vi "CarWashTest.vi"(0 "Wash Option":string, 2 "Label":string, 5 "Car Position":u8=1, 7 "Elapsed Time":dbl=5.0, 11 "error in":errorcluster) -> (15 "error out":errorcluster)   [LabVIEW 2016]
uses:
  Car Wash 16.0/Car Wash.vi
  main/apis/Stimulus/ValueSignalByPathString.vi
  main/apis/Assert/AssertControlValueCompare/AssertControlValueEqual.vi
  main/apis/Setup/GetVI/GetVIByPath.vi
  main/apis/Assert/AssertControlValueCompare/AssertControlValueAlmostEqual.vi
  <vilib>/addons/_JKI Toolkits/Caraya/classes/Test/Test.lvclass
  Car Wash 16.0/Car Wash.lvlib
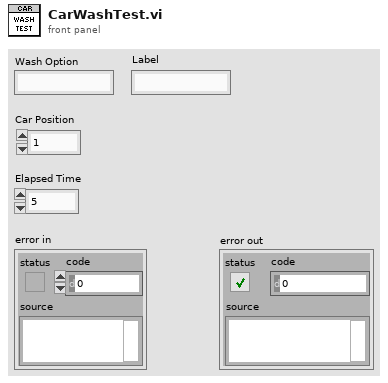
[diagram p1: front panel]
types:
  T1 = enum32{"Invalid", "Standard", "Closed", "Hidden", "Minimized", "Maximized"}
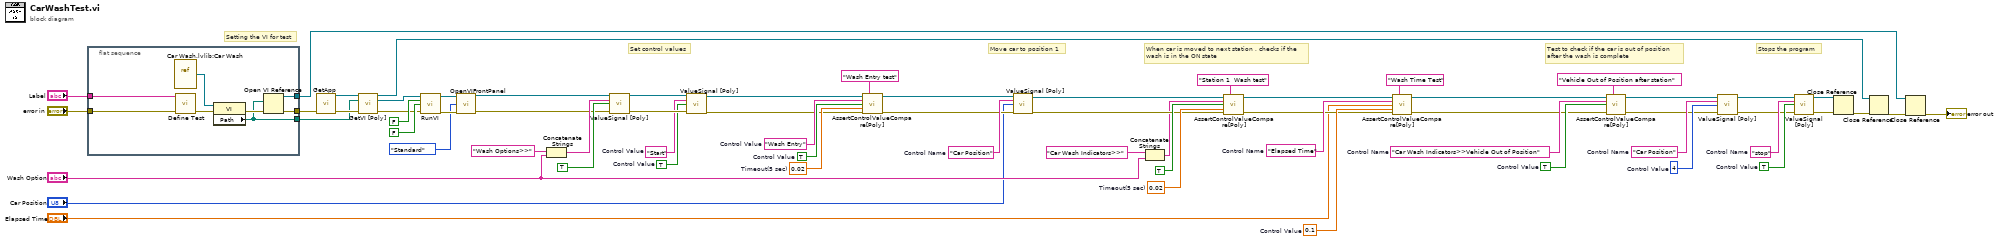
[diagram p0: block diagram]
diagram:
  w11 = TRUE  # Control Value
  w12 = "stop"  # Control Name
  w18 = "Start"  # Control Value
  w19 = TRUE  # Control Value
  w44 = u8 4  # Control Value
  w45 = "Car Position"  # Control Name
  w51 = TRUE  # Control Value
  w59 = 0.02  # Timeout(5 sec)
  w56 = 0.1  # Control Value
  w57 = "Elapsed Time"  # Control Name
  w52 = "Car Wash Indicators>>Vehicle Out of Position"  # Control Name
  w63 = "Car Position"  # Control Name
  w64 = 0.02  # Timeout(5 sec)
  w65 = TRUE  # Control Value
  w66 = "Wash Entry"  # Control Value
  # "Stops the program"
  # "Set control values"
  # "Setting the VI for test"
  # "Test to check if the car is out of position \nafter the wash is complete"
  # "When car is moved to next station , checks if the\nwash is in the ON state"
  # "Move car to position 1"
  n1 = flat-sequence {
    tunnel: [w71] -> w39
    tunnel: [w70] -> w2
    tunnel: [w69] -> w34
    tunnel: "error in" -> [w68]
    tunnel: "Label" -> [w67]
    frame #0 {
      n2 = vi-ref "Car Wash.lvlib:Car Wash.vi"() -> (w73:refnum<vi>)
      n3 = call <vilib>:"Define Test.vi"("error in (no error)"=w68, "Label (VI Title)"=w67) -> ("error out"=w74:errorcluster)  [unwired: 9 in]
      n4 = property on="Property Node" class="VI"(reference=w73, error in=w74) -> (error out=w72:errorcluster, "Path"=w69:path)  [unwired: 1 out]
      n5 = Open VI Reference(vi path=w69, error in (no error)=w72) -> (vi reference=w70:refnum<vi>, error out=w71:errorcluster)  [unwired: 4 in]
    }
  }
  n6 = call "GetApp.vi"("error in (no error)"=w39) -> ("Application Ref"=w35:refnum<vi>, "error out"=w36:errorcluster)  [unwired: 13 in]
  n7 = call-poly "GetVI [Poly].vi"("Application Ref in"=w35, "VI Path"=w34, "error in (no error)"=w36) -> ("Application Ref out"=w3:refnum<vi>, "VI Reference"=w33:refnum<vi>, "error out"=w32:errorcluster)  [unwired: 10 in]
  n8 = call "RunVI.vi"("VI Reference In"=w33, "Wait Until Done (F)"=FALSE ("Wait Until Done"), "Auto Dispose Reference (F)"=FALSE ("Auto Dispose Reference"), "error in"=w32) -> ("VI Reference Out"=w30:refnum<vi>, "error out"=w31:errorcluster)  [unwired: 10 in]
  n9 = call "OpenVIFrontPanel.vi"("VI Reference In"=w30, "State"=T1."Standard", "error in"=w31) -> ("VI Reference Out"=w22:refnum<vi>, "error out"=w27:errorcluster)  [unwired: 11 in]
  n10 = Concatenate Strings("Wash Options>>", "Wash Option") -> (w40:string)
  n11 = call-poly "ValueSignal [Poly].vi"("VI Reference In"=w22, "Control Name"=w40, "Value (Signaling)"=TRUE, "error in"=w27) -> ("VI Reference Out"=w23:refnum<vi>, "error out"=w25:errorcluster)  [unwired: 10 in]
  n12 = call-poly "ValueSignal [Poly].vi"("VI Reference In"=w23, "Control Name"=w18, "Value (Signaling)"=w19, "error in"=w25) -> ("VI Reference Out"=w20:refnum<vi>, "error out"=w24:errorcluster)  [unwired: 10 in]
  n13 = call-poly "AssertControlValueCompare[Poly].vi"("VI Reference In"=w20, "Label"="Wash Entry test", "Control Name"=w66, "Control Value"=w65, "Timeout(5 sec)"=w64, "error out"=w24) -> ("VI Reference Out"=w61:refnum<vi>, "error out"=w62:errorcluster)  [unwired: 8 in]
  n14 = call-poly "ValueSignal [Poly].vi"("VI Reference In"=w61, "Control Name"=w63, "Value (Signaling)"="Car Position", "error in"=w62) -> ("VI Reference Out"=w46:refnum<vi>, "error out"=w47:errorcluster)  [unwired: 10 in]
  n15 = Concatenate Strings("Car Wash Indicators>>", "Wash Option") -> (w16:string)
  n16 = call-poly "AssertControlValueCompare[Poly].vi"("VI Reference In"=w46, "Label"="Station 1  Wash test", "Control Name"=w16, "Control Value"=TRUE, "Timeout(5 sec)"=w59, "error out"=w47) -> ("VI Reference Out"=w54:refnum<vi>, "error out"=w55:errorcluster)  [unwired: 8 in]
  n17 = call-poly "AssertControlValueCompare[Poly].vi"("VI Reference In"=w54, "Label"="Wash Time Test", "Control Name"=w57, "Control Value"="Elapsed Time", "Tolerance"=w56, "error out"=w55) -> ("VI Reference Out"=w48:refnum<vi>, "error out"=w49:errorcluster)  [unwired: 8 in]
  n18 = call-poly "AssertControlValueCompare[Poly].vi"("VI Reference In"=w48, "Label"="Vehicle Out of Position after station", "Control Name"=w52, "Control Value"=w51, "error out"=w49) -> ("VI Reference Out"=w43:refnum<vi>, "error out"=w42:errorcluster)  [unwired: 9 in]
  n19 = call-poly "ValueSignal [Poly].vi"("VI Reference In"=w43, "Control Name"=w45, "Value (Signaling)"=w44, "error in"=w42) -> ("VI Reference Out"=w4:refnum<vi>, "error out"=w5:errorcluster)  [unwired: 10 in]
  n20 = call-poly "ValueSignal [Poly].vi"("VI Reference In"=w4, "Control Name"=w12, "Value (Signaling)"=w11, "error in"=w5) -> ("VI Reference Out"=w8:refnum<vi>, "error out"=w10:errorcluster)  [unwired: 10 in]
  n21 = Close Reference(reference=w8, error in (no error)=w10) -> (error out=w9:errorcluster)
  n22 = Close Reference(reference=w3, error in (no error)=w9) -> (error out=w7:errorcluster)
  n23 = Close Reference(reference=w2, error in (no error)=w7) -> (error out=→"error out":errorcluster)
